vi "Create State Transition Map.vi"(8 "error in (no error)":errorcluster, 10 "Transition Map in":T1(array[cluster]), 11 "StateMachine in":refnum<class "StateMachine.lvclass">) -> (0 "error out":errorcluster, 2 "Empty transitions?":bool, 3 "StateMachine out":refnum<class "StateMachine.lvclass">)   [LabVIEW 2019, in "State Machine.lvlib" / "StateMachine.lvclass"]
uses:
  StateMachine.lvclass
  StateMachine.lvclass/StateMachine.ctl
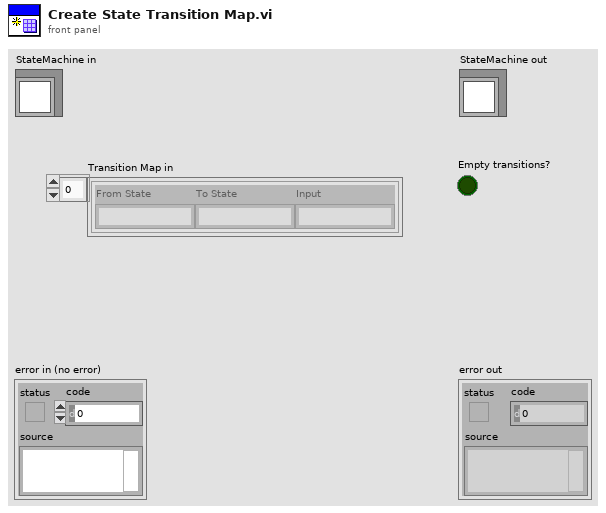
[diagram p1: front panel]
types:
  T1 = cluster{"From State":string, "To State":string, "Input":string}[]
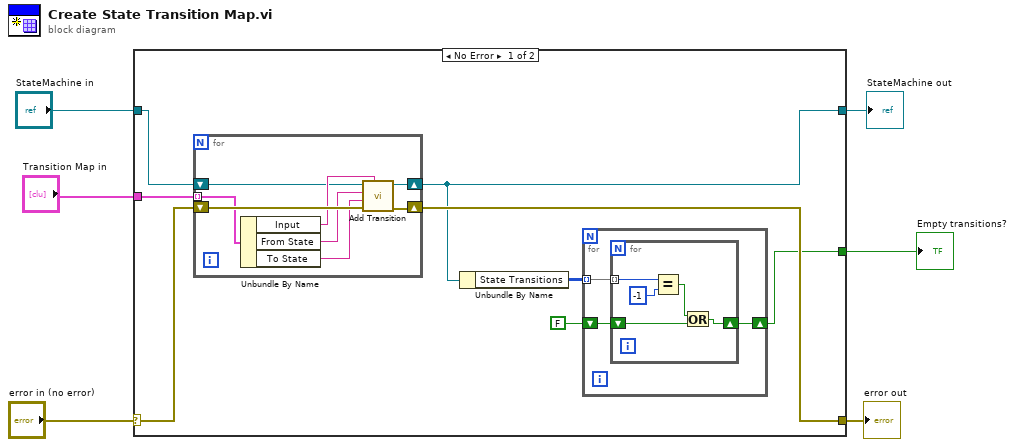
[diagram p0: block diagram]
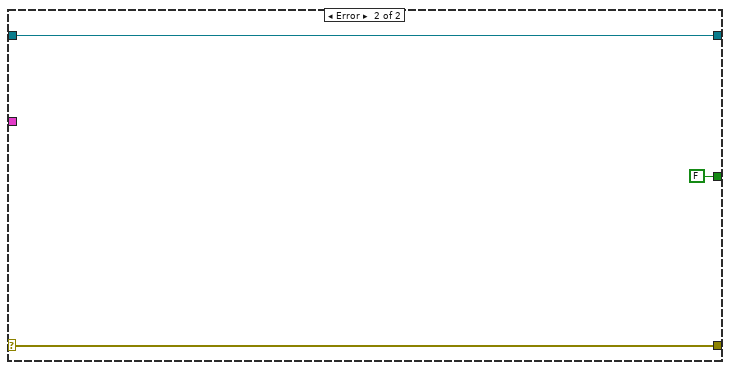
[diagram p2: hidden frame]
diagram:
  n1 = case shown="No Error" "error in (no error)" {
    selector: "error in (no error)" -> [w12 w33]
    tunnel: [w13 w33] -> w5
    tunnel: [w10 w32] -> w3
    tunnel: "StateMachine in" -> [w14 w32]
    tunnel: "Transition Map in" -> [w11 _]
    tunnel: [w7 FALSE] -> w1
    frame No Error {
      n2 = for {
        tunnel: w11 -> [w28] mode=indexing
        shift-right: [w23] -> w10
        shift-left: w14 -> [w24]
        shift-right: [w29] -> w13
        shift-left: w12 -> [w30]
        n3 = Unbundle By Name(w28) -> ("Input"=w27:string, "From State"=w26:string, "To State"=w25:string)
        n4 = call-dynamic "Add Transition.vi"("Input"=w27, "error in (no error)"=w30, "To State"=w25, "From State"=w26, "StateMachine in"=w24) -> ("error out"=w29:errorcluster, "StateMachine out"=w23:refnum<class "StateMachine.lvclass">)  [unwired: 5 in]
      }
      n5 = Unbundle By Name(w10) -> ("State Transitions"=w9:i32[][])
      n6 = for {
        tunnel: w9 -> [w17] mode=indexing
        shift-right: [w15] -> w7
        shift-left: FALSE -> [w16]
        n7 = for {
          tunnel: w17 -> [w20] mode=indexing
          shift-right: [w21] -> w15
          shift-left: w16 -> [w22]
          n8 = Equal?(x=w20, y=-1) -> (x = y?=w19:bool)
          n9 = Or(x=w19, y=w22) -> (x .or. y?=w21:bool)
        }
      }
    }
    frame Error {
    }
  }
  "error out" <- w5
  "StateMachine out" <- w3
  "Empty transitions?" <- w1
